vi "ex14-5.vi"() -> ()   [LabVIEW 2014]
uses:
  <vilib>/NXT/Subs/MotorOutput.ctl
  <vilib>/NXT/Dual Mode Library/prims/inRangeAndCoerce/inRangeAndCoerce_float.vi
  <vilib>/NXT/Dual Mode Library/Motors/MotorDistance_Single.vi
panel:
  out "2^0":bool
  out "2^1":bool
  out "2^2":bool
  out "2^3":bool
  out "2^4":bool
  out "2^5":bool
  out "2^6":bool
  out "2^7":bool
  out "2^8":bool
  out "2^9":bool
  out "2^10":bool
  out "2^11":bool
  out "2^12":bool
  out "2^13":bool
  out "2^14":bool
  out "2^15":bool
  out "溢位?65536":bool
  in  "輸入":dbl
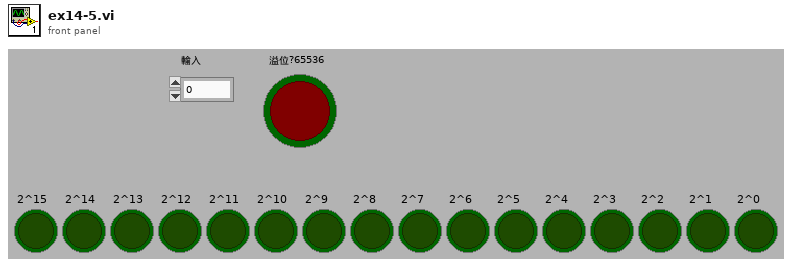
[diagram p1: front panel]
types:
  T1 = typedef "MotorOutput.ctl" = u8
  T2 = typedef "LVHSConnector.ctl" = refnum<class "BrickReference.lvclass">
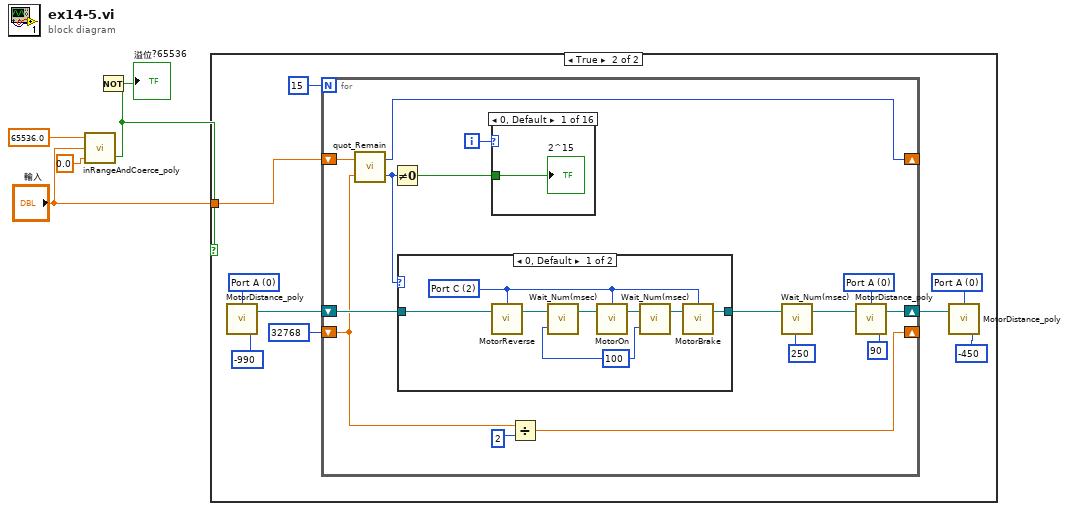
[diagram p0: block diagram]
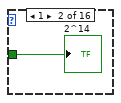
[diagram p3: hidden frame]
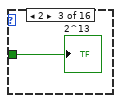
[diagram p4: hidden frame]
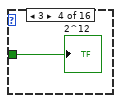
[diagram p5: hidden frame]
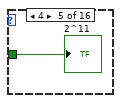
[diagram p6: hidden frame]
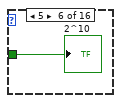
[diagram p7: hidden frame]
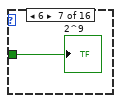
[diagram p8: hidden frame]
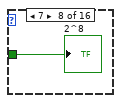
[diagram p9: hidden frame]
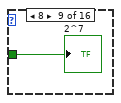
[diagram p10: hidden frame]
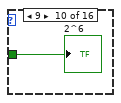
[diagram p11: hidden frame]
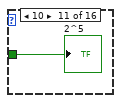
[diagram p12: hidden frame]
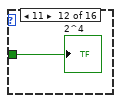
[diagram p13: hidden frame]
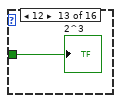
[diagram p14: hidden frame]
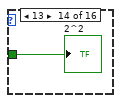
[diagram p15: hidden frame]
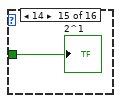
[diagram p16: hidden frame]
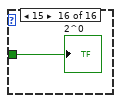
[diagram p17: hidden frame]
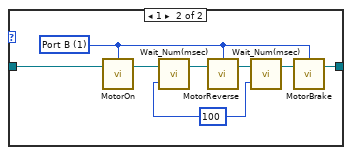
[diagram p18: hidden frame]
diagram:
  n1 = call-poly <vilib>:"inRangeAndCoerce_poly.vi"("lower limit"=0.0, "x"="輸入", "upper limit"=65536.0 ("y")) -> ("In Range?"=w4:bool)  [unwired: 1 out]
  n2 = Not(x=w4) -> (.not. x?=→"溢位?65536":bool)
  n3 = case shown="True" w4 {
    tunnel: "輸入" -> [_ w13]
    frame False {
    }
    frame True {
      w6 = T1 0 items=["Port A", "Port B", "Port C", "All Ports"] ("Output Port (All Ports)")
      w7 = T1 0 items=["Port A", "Port B", "Port C", "All Ports"] ("Output Port (All Ports)")
      n4 = call-poly <vilib>:"MotorDistance_poly.vi"("Angle of Rotation (360)"=-990 ("Distance (100)"), "Output Port (All Ports)"=w7) -> ("NXT/EV3"=w11:T2)  [unwired: 2 in]
      n5 = for {
        N: 15 -> [_]
        shift-right: [w15] -> _
        shift-left: w13 -> [w21]
        shift-right: [w28] -> _
        shift-left: 32768 -> [w20]
        shift-right: [w25] -> w10
        shift-left: w11 -> [w27]
        i -> [w19]
        w16 = T1 0 items=["Port A", "Port B", "Port C", "All Ports"] ("Output Port (All Ports)")
        n6 = call <vilib>:"quot_Remain.vi"("y"=w20, "x"=w21) -> ("floor(x/y)"=w17:i32, "x-y*floor(x/y)"=w15:i32)
        n7 = Not Equal To 0?(x=w17) -> (x != 0?=w18:bool)
        n8 = case shown="0, Default" w17 {
          tunnel: w27 -> [w49 w56]
          tunnel: [w50 w55] -> w24
          frame 0, Default {
            w51 = u32 100 ("Time (100 msec)")
            w53 = T1 2 items=["Port A", "Port B", "Port C", "All Ports"] ("Output Port (All Ports)")
            n9 = call <vilib>:"MotorReverse.vi"("NXT/EV3"=w49, "Output Port (All Ports)"=w53) -> ("NXT/EV3"=w48:T2)  [unwired: 2 in]
            n10 = call <vilib>:"Wait_Num(msec).vi"("Time (100 msec)"=w51, "NXT/EV3"=w48) -> ("NXT/EV3"=w47:T2)  [unwired: 2 in]
            n11 = call <vilib>:"MotorOn.vi"("NXT/EV3"=w47, "Output Port (All Ports)"=w53) -> ("NXT/EV3"=w46:T2)  [unwired: 2 in]
            n12 = call <vilib>:"Wait_Num(msec).vi"("Time (100 msec)"=w51, "NXT/EV3"=w46) -> ("NXT/EV3"=w52:T2)  [unwired: 2 in]
            n13 = call <vilib>:"MotorBrake.vi"("NXT/EV3"=w52, "Port (All Ports)"=w53) -> ("NXT/EV3"=w50:T2)  [unwired: 2 in]
          }
          frame 1 {
            w54 = u32 100 ("Time (100 msec)")
            w61 = T1 1 items=["Port A", "Port B", "Port C", "All Ports"] ("Output Port (All Ports)")
            n14 = call <vilib>:"MotorOn.vi"("NXT/EV3"=w56, "Output Port (All Ports)"=w61) -> ("NXT/EV3"=w57:T2)  [unwired: 2 in]
            n15 = call <vilib>:"Wait_Num(msec).vi"("Time (100 msec)"=w54, "NXT/EV3"=w57) -> ("NXT/EV3"=w58:T2)  [unwired: 2 in]
            n16 = call <vilib>:"MotorReverse.vi"("NXT/EV3"=w58, "Output Port (All Ports)"=w61) -> ("NXT/EV3"=w59:T2)  [unwired: 2 in]
            n17 = call <vilib>:"Wait_Num(msec).vi"("Time (100 msec)"=w54, "NXT/EV3"=w59) -> ("NXT/EV3"=w60:T2)  [unwired: 2 in]
            n18 = call <vilib>:"MotorBrake.vi"("NXT/EV3"=w60, "Port (All Ports)"=w61) -> ("NXT/EV3"=w55:T2)  [unwired: 2 in]
          }
        }
        n19 = case shown="0, Default" w19 {
          tunnel: w18 -> [w30 w31 w32 w33 w34 w35 w36 w37 w38 w39 w40 w41 w42 w43 w44 w45]
          frame 0, Default {
            "2^15" <- w30
          }
          frame 1 {
            "2^14" <- w31
          }
          frame 2 {
            "2^13" <- w32
          }
          frame 3 {
            "2^12" <- w33
          }
          frame 4 {
            "2^11" <- w34
          }
          frame 5 {
            "2^10" <- w35
          }
          frame 6 {
            "2^9" <- w36
          }
          frame 7 {
            "2^8" <- w37
          }
          frame 8 {
            "2^7" <- w38
          }
          frame 9 {
            "2^6" <- w39
          }
          frame 10 {
            "2^5" <- w40
          }
          frame 11 {
            "2^4" <- w41
          }
          frame 12 {
            "2^3" <- w42
          }
          frame 13 {
            "2^2" <- w43
          }
          frame 14 {
            "2^1" <- w44
          }
          frame 15 {
            "2^0" <- w45
          }
        }
        n20 = Divide(x=w20, y=2) -> (x/y=w28:dbl)
        n21 = call <vilib>:"Wait_Num(msec).vi"("Time (100 msec)"=u32 250, "NXT/EV3"=w24) -> ("NXT/EV3"=w23:T2)  [unwired: 2 in]
        n22 = call-poly <vilib>:"MotorDistance_poly.vi"("Angle of Rotation (360)"=90 ("Distance (100)"), "NXT/EV3"=w23, "Output Port (All Ports)"=w16) -> ("NXT/EV3"=w25:T2)  [unwired: 1 in]
      }
      n23 = call-poly <vilib>:"MotorDistance_poly.vi"("Angle of Rotation (360)"=-450 ("Distance (100)"), "NXT/EV3"=w10, "Output Port (All Ports)"=w6) -> ()  [unwired: 1 in, 1 out]
    }
  }
